vi "ConvertBooleanToSCPIValue.vi"(11 "Boolean":bool) -> (3 "SCPI Value":string)   [LabVIEW 2012, in "Keithley-6485.lvlib"]
uses:
  Keithley-6485.lvlib
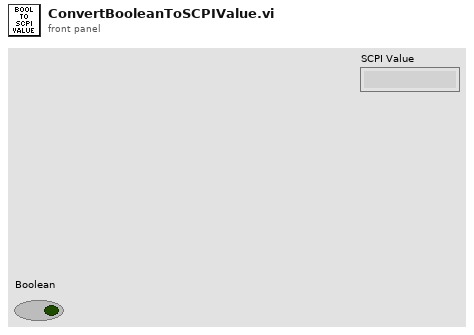
[diagram p1: front panel]
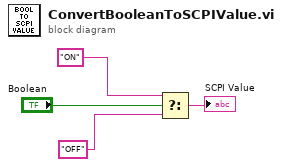
[diagram p0: block diagram]
diagram:
  n1 = Select(t="ON", s="Boolean", f="OFF") -> (s? t:f=→"SCPI Value":string)
